vi "sqlconfig.vi"(11 "路径":path) -> (0 "db":string, 1 "psw":string, 2 "user":string, 3 "ip":string, 4 "table_D2":string, 5 "table_M2":string, 6 "table_D1":string, 7 "table_M1":string)   [LabVIEW 2011]
panel:
  out "文本":string
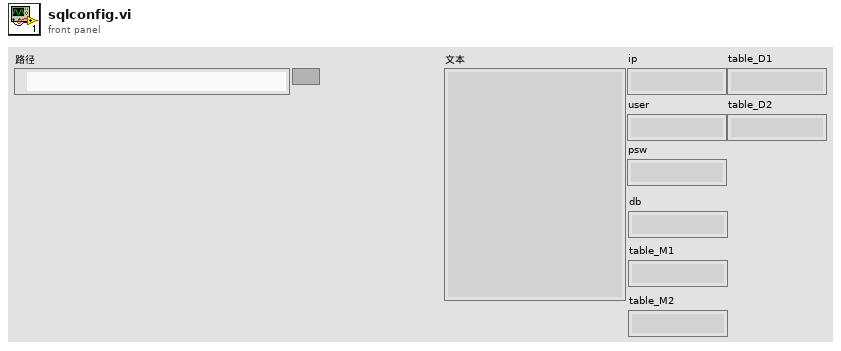
[diagram p1: front panel]
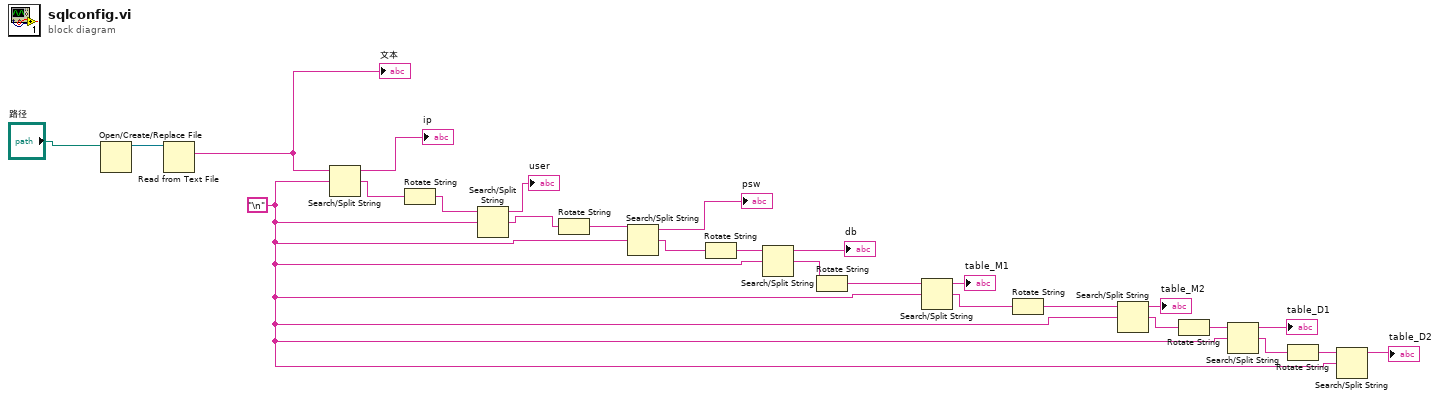
[diagram p0: block diagram]
diagram:
  w2 = "\n"
  n1 = Open/Create/Replace File(file path (use dialog)="路径") -> (refnum out=w25:refnum<file>)  [unwired: 5 in, 2 out]
  n2 = Read from Text File(file (use dialog)=w25) -> (text=w24:string)  [unwired: 3 in, 3 out]
  "文本" <- w24
  n3 = Search/Split String(string=w24, search string/char (-)=w2) -> (substring before match=→"ip":string, match + rest of string=w22:string)  [unwired: 1 in, 1 out]
  n4 = Rotate String(1:w22) -> (0:w21:string)
  n5 = Search/Split String(string=w21, search string/char (-)=w2) -> (substring before match=→"user":string, match + rest of string=w19:string)  [unwired: 1 in, 1 out]
  n6 = Rotate String(1:w19) -> (0:w18:string)
  n7 = Search/Split String(string=w18, search string/char (-)=w2) -> (substring before match=→"psw":string, match + rest of string=w16:string)  [unwired: 1 in, 1 out]
  n8 = Rotate String(1:w16) -> (0:w15:string)
  n9 = Search/Split String(string=w15, search string/char (-)=w2) -> (substring before match=→"db":string, match + rest of string=w13:string)  [unwired: 1 in, 1 out]
  n10 = Rotate String(1:w13) -> (0:w12:string)
  n11 = Search/Split String(string=w12, search string/char (-)=w2) -> (substring before match=→"table_M1":string, match + rest of string=w8:string)  [unwired: 1 in, 1 out]
  n12 = Rotate String(1:w8) -> (0:w9:string)
  n13 = Search/Split String(string=w9, search string/char (-)=w2) -> (substring before match=→"table_M2":string, match + rest of string=w7:string)  [unwired: 1 in, 1 out]
  n14 = Rotate String(1:w7) -> (0:w6:string)
  n15 = Search/Split String(string=w6, search string/char (-)=w2) -> (substring before match=→"table_D1":string, match + rest of string=w4:string)  [unwired: 1 in, 1 out]
  n16 = Rotate String(1:w4) -> (0:w3:string)
  n17 = Search/Split String(string=w3, search string/char (-)=w2) -> (substring before match=→"table_D2":string)  [unwired: 1 in, 2 out]
